vi "Delete Bucket Policy.vi"(8 "error in (no error)":errorcluster, 9 "Bucket":string) -> (0 "error out":errorcluster)   [LabVIEW 2011, in "LV Interface for Amazon S3.lvlib"]
doc: "<B>Removes the Policy</B> on a specified <B>Bucket</B>. To use the operation, you <B>must have DeletePolicy permission</B> on the specified bucket and have to <B>be the bucket owner</B>."
uses:
  LV Interface for Amazon S3.lvlib
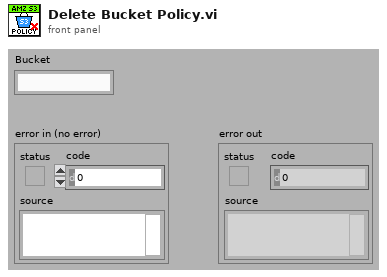
[diagram p1: front panel]
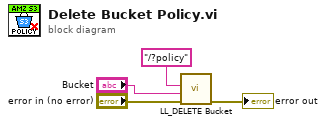
[diagram p0: block diagram]
diagram:
  n1 = call "LL_DELETE Bucket.vi"("error in (no error)"="error in (no error)", "Bucket"="Bucket", "Path and query string"="/?policy") -> ("error out"=→"error out":errorcluster)  [unwired: 7 in, 1 out]
